vi "Get Scanner.vi"(8 "error in (no error)":errorcluster, 11 "Pulse Gating System (HV supply) in":refnum<class "Pulse Gating System (HV supply).lvclass">) -> (0 "error out":errorcluster, 2 "Default Scanner out":refnum<class "Scanner.lvclass">)   [LabVIEW 2023, in "Pulse Gating System (HV supply).lvclass"]
doc: "(Dynamic) Returns the default Scanner object that scans over this Scannable. (Note that a Scannable may have multiple Scanners associated with it.) A Scanner is an analogue to an Iterator class in other languages."
uses:
  Pulse Gating System (HV supply).lvclass
  Scanners/Scanner/Scanner.lvclass
  Scanners/Voltage Pulse Gating System (HV supply)/Voltage Pulse Gating System (HV supply).lvclass
  C:/LabVIEW-programs/Scanners/Scanner/Scanner.lvclass
  Utility Classes/Scannable/Scannable.lvclass
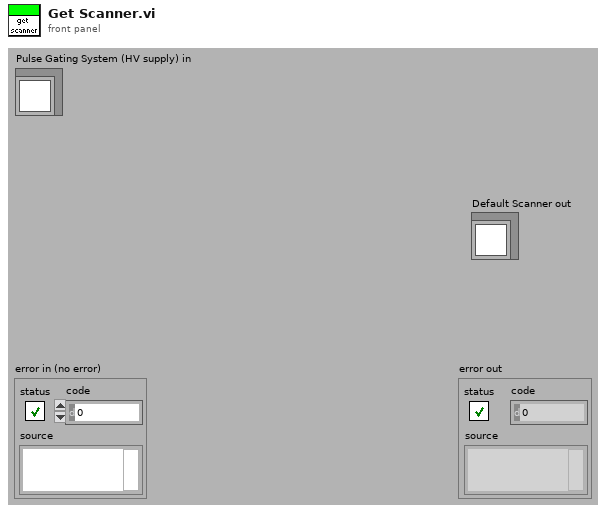
[diagram p1: front panel]
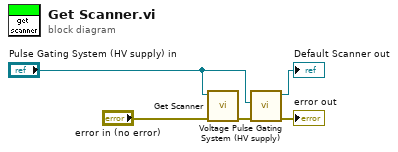
[diagram p0: block diagram]
diagram:
  n1 = call-parent "Get Scanner.vi"("error in (no error)"="error in (no error)", "Scannable in"="Pulse Gating System (HV supply) in") -> ("error out"=w2:errorcluster)  [unwired: 8 in, 1 out]
  n2 = call "Voltage Pulse Gating System (HV supply).vi"("error in (no error)"=w2, "Pulse Gating System (HV supply).lvclass"="Pulse Gating System (HV supply) in") -> ("error out"=→"error out":errorcluster, "Voltage Pulse Gating System (HV supply) out"=→"Default Scanner out":refnum<class "Voltage Pulse Gating System (HV supply).lvclass">)  [unwired: 8 in]
